vi "Scan.vi"(8 "error in":errorcluster, 10 "Scan Measurement (on)":enum16{"off", "on"}(ring)=enum."on", 11 "VISA resource name":refnum<visa-resource-name>) -> (0 "error out":errorcluster, 3 "VISA resource name out":refnum<visa-resource-name>)   [LabVIEW 2019, in "Andeen-Hagerling 2700(400 firmware).lvlib"]
doc: "Initiates or discontinues scan parameter measurements which are taken continuously, one after another."
uses:
  Andeen-Hagerling 2700(400 firmware).lvlib
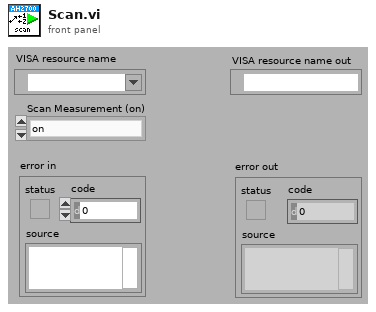
[diagram p1: front panel]
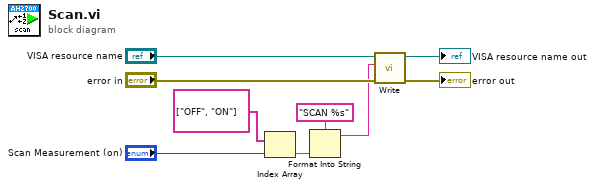
[diagram p0: block diagram]
diagram:
  n1 = Index Array(array=string[] ["OFF", "ON"], index="Scan Measurement (on)") -> (element=w2:string)
  n2 = Format Into String(format string="SCAN %s", w2) -> (resulting string=w1:string)  [unwired: 2 in, 1 out]
  n3 = call "Write.vi"("error in"="error in", "command"=w1, "VISA resource name"="VISA resource name") -> ("error out"=→"error out":errorcluster, "VISA resource name out"=→"VISA resource name out":refnum<visa-resource-name>)  [unwired: 7 in]
